vi "Send move to stages.vi"(8 "error in (no error)":errorcluster, 11 "Tomo in":refnum<class "Tomo.lvclass">) -> (0 "error out":errorcluster, 3 "Tomo out":refnum<class "Tomo.lvclass">)   [LabVIEW 2012, in "Tomo.lvclass"]
uses:
  Tomo.lvclass
  <vilib>/Distrio/Murmex/GenericMessage/GenericMessage.lvclass
  <vilib>/Distrio/Murmex/StartMessage/StartMessage.lvclass
  <vilib>/Distrio/Murmex/Message/Message.lvclass
  <vilib>/Distrio/Murmex/Murmex/Murmex.lvclass
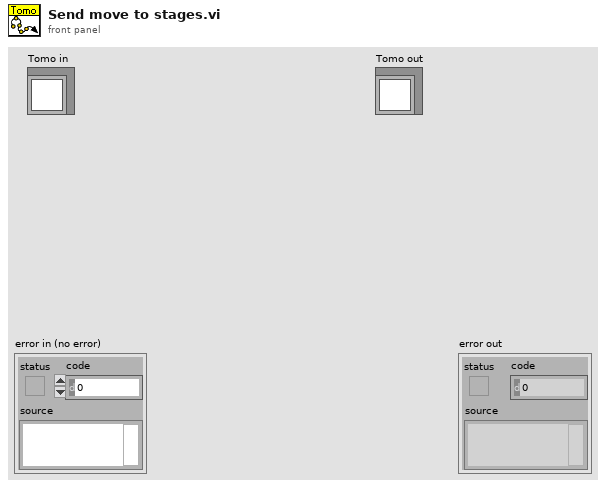
[diagram p1: front panel]
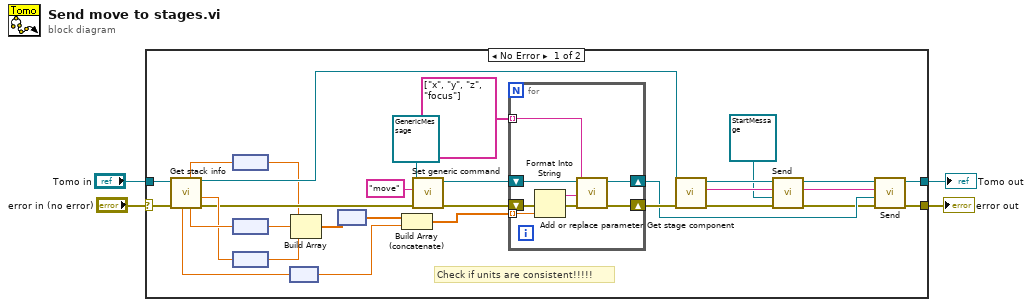
[diagram p0: block diagram]
diagram:
  n1 = case shown="No Error" "error in (no error)" {
    selector: "error in (no error)" -> [w31 w44]
    tunnel: [w22 w44] -> w3
    tunnel: [w23 w43] -> w2
    tunnel: "Tomo in" -> [w32 w43]
    frame No Error {
      # "Check if units are consistent!!!!!"
      n2 = call-dynamic "Get stack info.vi"("error in (no error)"=w31, "Tomo in"=w32) -> ("error out"=w18:errorcluster, "Z start"=w28:dbl, "Tomo out"=w17:refnum<class "Tomo.lvclass">, "Y position"=w29:dbl, "X position"=w30:dbl, "Default focus"=w6:dbl[unit])  [unwired: 3 in, 1 out]
      n3 = node(w30) -> (w14:dbl[unit])
      n4 = node(w29) -> (w16:dbl[unit])
      n5 = node(w28) -> (w15:dbl[unit])
      n6 = node(w6) -> (w5:dbl)
      n7 = Build Array(w14, w16, w15) -> (w24:dbl[unit][])
      n8 = node(w24) -> (w19:dbl[])
      n9 = Build Array (concatenate)(w19, w5) -> (w7:dbl[])
      n10 = call <vilib>:"Set generic command.vi"("error in (no error)"=w18, "generic command"="move" ("command string"), "GenericMessage in"=refnum<class "GenericMessage.lvclass"> refnum ("Murmex.lvlib:GenericMessage")) -> ("error out"=w27:errorcluster, "GenericMessage out"=w26:refnum<class "GenericMessage.lvclass">)  [unwired: 7 in]
      n11 = for {
        shift-right: [w36] -> w21
        shift-left: w27 -> [w42]
        shift-right: [w37] -> w20
        shift-left: w26 -> [w41]
        tunnel: string[] ["x", "y", "z", "focus"] -> [w39] mode=indexing
        tunnel: w7 -> [w38] mode=indexing
        n12 = Format Into String(error in=w42, w38) -> (resulting string=w35:string, error out=w40:errorcluster)  [unwired: 2 in]
        n13 = call <vilib>:"Add or replace parameter.vi"("error in (no error)"=w40, "value"=w35, "name"=w39, "Message in"=w41) -> ("error out"=w36:errorcluster, "Message out"=w37:refnum<class "GenericMessage.lvclass">)  [unwired: 6 in]
      }
      n14 = call-dynamic "Get stage component.vi"("error in (no error)"=w21, "Tomo in"=w17) -> ("error out"=w13:errorcluster, "stage component"=w9:string, "Tomo out"=w11:refnum<class "Tomo.lvclass">)  [unwired: 7 in]
      n15 = call <vilib>:"Send.vi"("error in (no error)"=w13, "Message"=refnum<class "StartMessage.lvclass"> refnum ("Distrio Murmex 1.1:StartMessage"), "recipient"=w9, "Murmex in"=w11) -> ("error out"=w12:errorcluster, "Murmex out"=w10:refnum<class "Tomo.lvclass">)  [unwired: 6 in]
      n16 = call <vilib>:"Send.vi"("error in (no error)"=w12, "Message"=w20, "recipient"=w9, "Murmex in"=w10) -> ("error out"=w22:errorcluster, "Murmex out"=w23:refnum<class "Tomo.lvclass">)  [unwired: 6 in]
    }
    frame Error {
    }
  }
  "error out" <- w3
  "Tomo out" <- w2
